vi "显示特定位置.vi"(10 "条码编号":string[](array[string]), 11 "MulticolumnListbox输入":refnum<vi>) -> (2 "数组输出":string[][](array[string]), 3 "MulticolumnListbox输出":refnum<vi>)   [LabVIEW 2011]
uses:
  <vilib>/Utility/miscctls.llb/LVRowAndColumnTypeDef.ctl
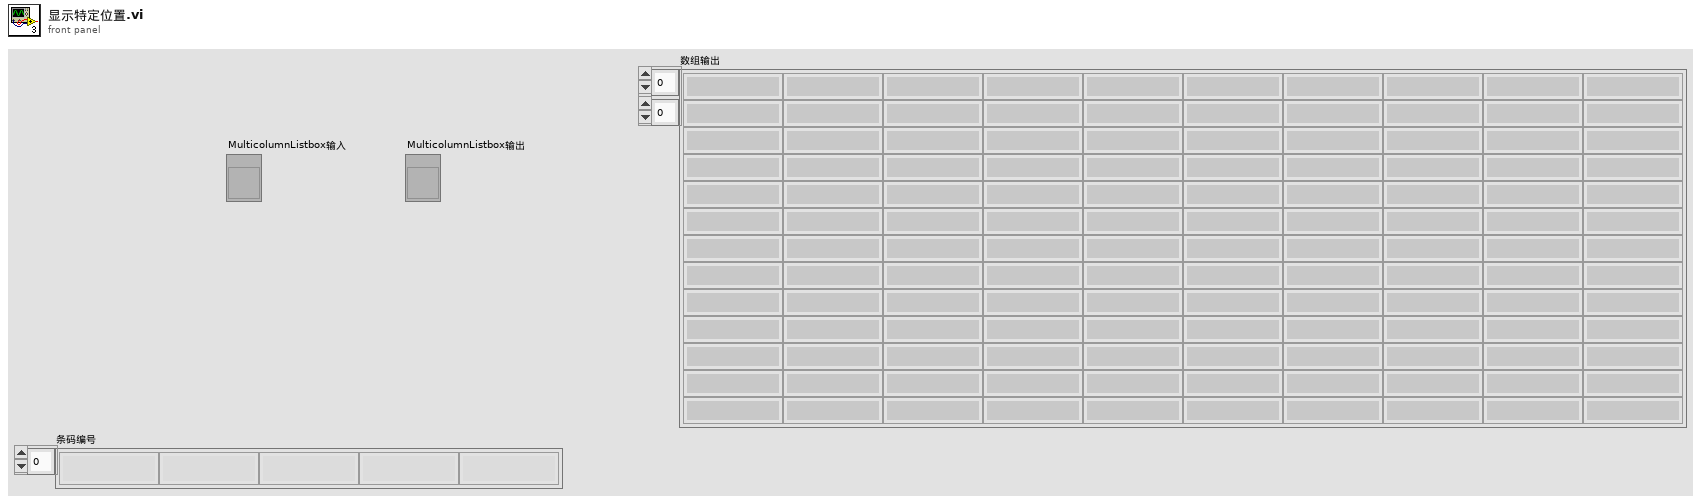
[diagram p1: front panel]
types:
  T1 = typedef "LVRowAndColumnTypeDef.ctl" = cluster{"Row":i32, "Column":i32}
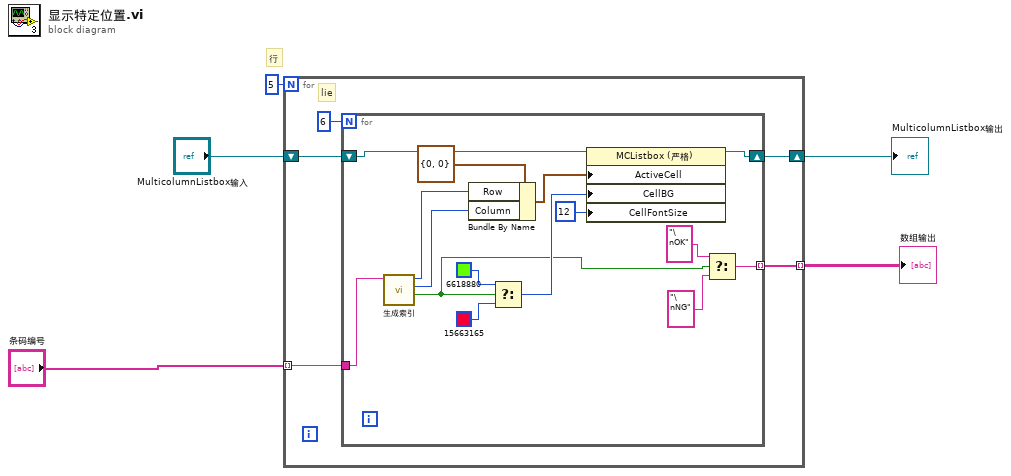
[diagram p0: block diagram]
diagram:
  # "行"
  n1 = for {
    N: 5 -> [_]
    shift-right: [w9] -> w5
    shift-left: "MulticolumnListbox输入" -> [w10]
    tunnel: [w8] -> w3 mode=indexing
    tunnel: "条码编号" -> [w6] mode=indexing
    # "lie"
    n2 = for {
      N: 6 -> [_]
      shift-right: [w24] -> w9
      shift-left: w10 -> [w25]
      tunnel: [w21] -> w8 mode=indexing
      tunnel: w6 -> [w20]
      n3 = call "生成索引.vi"("data out输入"=w20) -> ("OK"=w14:bool, "行"=w18:i32, "列"=w19:i32)  [unwired: 8 in]
      n4 = Bundle By Name(cluster=T1 {"Row"=0, "Column"=0} ("活动单元格:活动单元格"), "Row"=w19, "Column"=w18) -> (w12:T1)
      n5 = Select(t=u32 6618880, s=w14, f=u32 15663165) -> (s? t:f=w15:u32)
      n6 = property class="MCListbox (严格)"(reference=w25, "ActiveCell"=w12, "CellBG"=w15, "CellFontSize"=u32 12 ("活动单元格:单元格字体:字号")) -> (reference out=w24:refnum<vi>)  [unwired: 1 in, 1 out]
      n7 = Select(t="\nOK", s=w14, f="\nNG") -> (s? t:f=w21:string)
    }
  }
  "MulticolumnListbox输出" <- w5
  "数组输出" <- w3
